vi "find_target_pose.vi"(10 "points":dbl[][](array[numeric]) format="%#.0f") -> (2 "Result":T1 format="%#_3f")   [LabVIEW 2013]
uses:
  <vilib>/Analysis/Matrix/Datatypes/RealMatrix.ctl
  <vilib>/Analysis/Matrix/Numeric/Conversions/Array To Matrix - RA.vi
  utilities/labview/norm_vec.vi
  <vilib>/Analysis/Matrix/NI_Matrix.lvlib
panel:
  out "+y":dbl[](array[numeric]) format="%#.0f"
  out "+x":dbl[](array[numeric]) format="%#.0f"
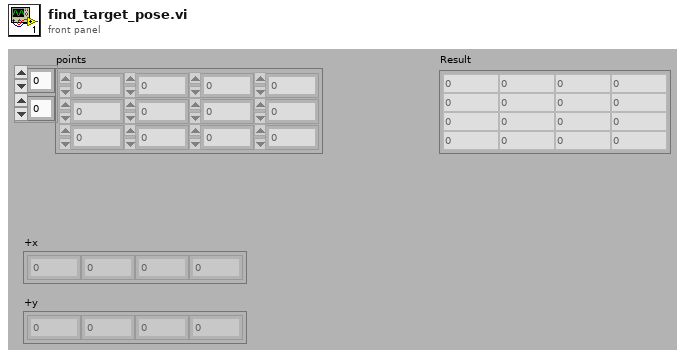
[diagram p1: front panel]
types:
  T1 = typedef "NI_Matrix.lvlib/RealMatrix.ctl" = dbl[][]
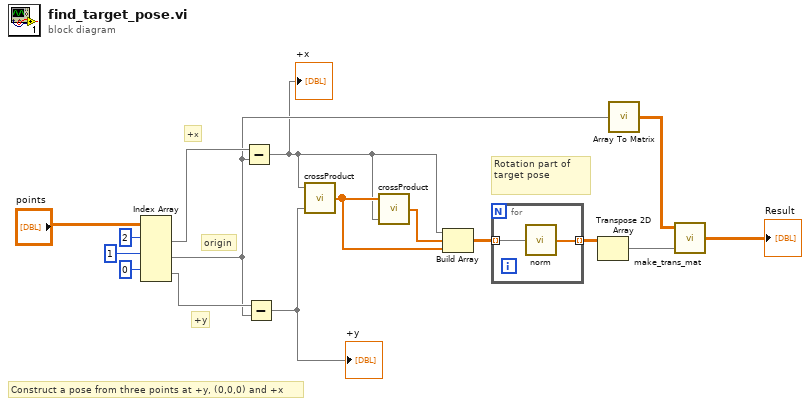
[diagram p0: block diagram]
diagram:
  # "Construct a pose from three points at +y, (0,0,0) and +x"
  # "Rotation part of target pose"
  # "+y"
  # "origin"
  # "+x"
  n1 = Index Array(array="points", index (row) #1=2 ("index (row)"), index (row) #2=1 ("index (row)"), index (row) #3=0 ("index (row)")) -> (element #1=w12:dbl[], element #2=w4:dbl[], element #3=w11:dbl[])  [unwired: 3 in]
  n2 = Subtract(x=w12, y=w4) -> (x-y=w1:dbl[])
  "+x" <- w1
  n3 = Subtract(x=w11, y=w4) -> (x-y=w2:dbl[])
  "+y" <- w2
  n4 = call "crossProduct.vi"("B"=w2, "A"=w1) -> ("A x B"=w8:dbl[])  [unwired: 3 out]
  n5 = call "crossProduct.vi"("B"=w1, "A"=w8) -> ("A x B"=w7:dbl[])  [unwired: 3 out]
  n6 = Build Array(w1, w7, w8) -> (w10:dbl[][])
  n7 = for {
    tunnel: w10 -> [w18] mode=indexing
    tunnel: [w17] -> w9 mode=indexing
    n8 = call-poly "norm.vi"("vector"=w18) -> ("normalized vector"=w17:dbl[])  [unwired: 4 out]
  }
  n9 = Transpose 2D Array(2D array=w9) -> (transposed array=w6:dbl[][])
  n10 = call-poly <vilib>:"Array To Matrix.vi"("Real 1D Array"=w4) -> ("Real Matrix (Column Vector)"=w5:T1)
  n11 = call "make_trans_mat.vi"("Rotation"=w6, "Translation"=w5) -> ("Transform"=→"Result":T1)  [unwired: 3 out]
